vi "Write Read Visa Port Waitfor.vi"(6 "Wait for timeout (secs)":dbl=10.0, 7 "Wait for in RX":string, 8 "error in (no error)":errorcluster, 9 "Wait for read Msecs":dbl=500.0, 10 "write buffer":string, 11 "VISA Refnum in":refnum<visa-resource-name>) -> (0 "error out":errorcluster, 1 "Elapsed Time":string, 2 "read buffer":string, 3 "VISA resource name out":refnum<visa-resource-name>)   [LabVIEW 2013]
panel:
  in  "stop":bool
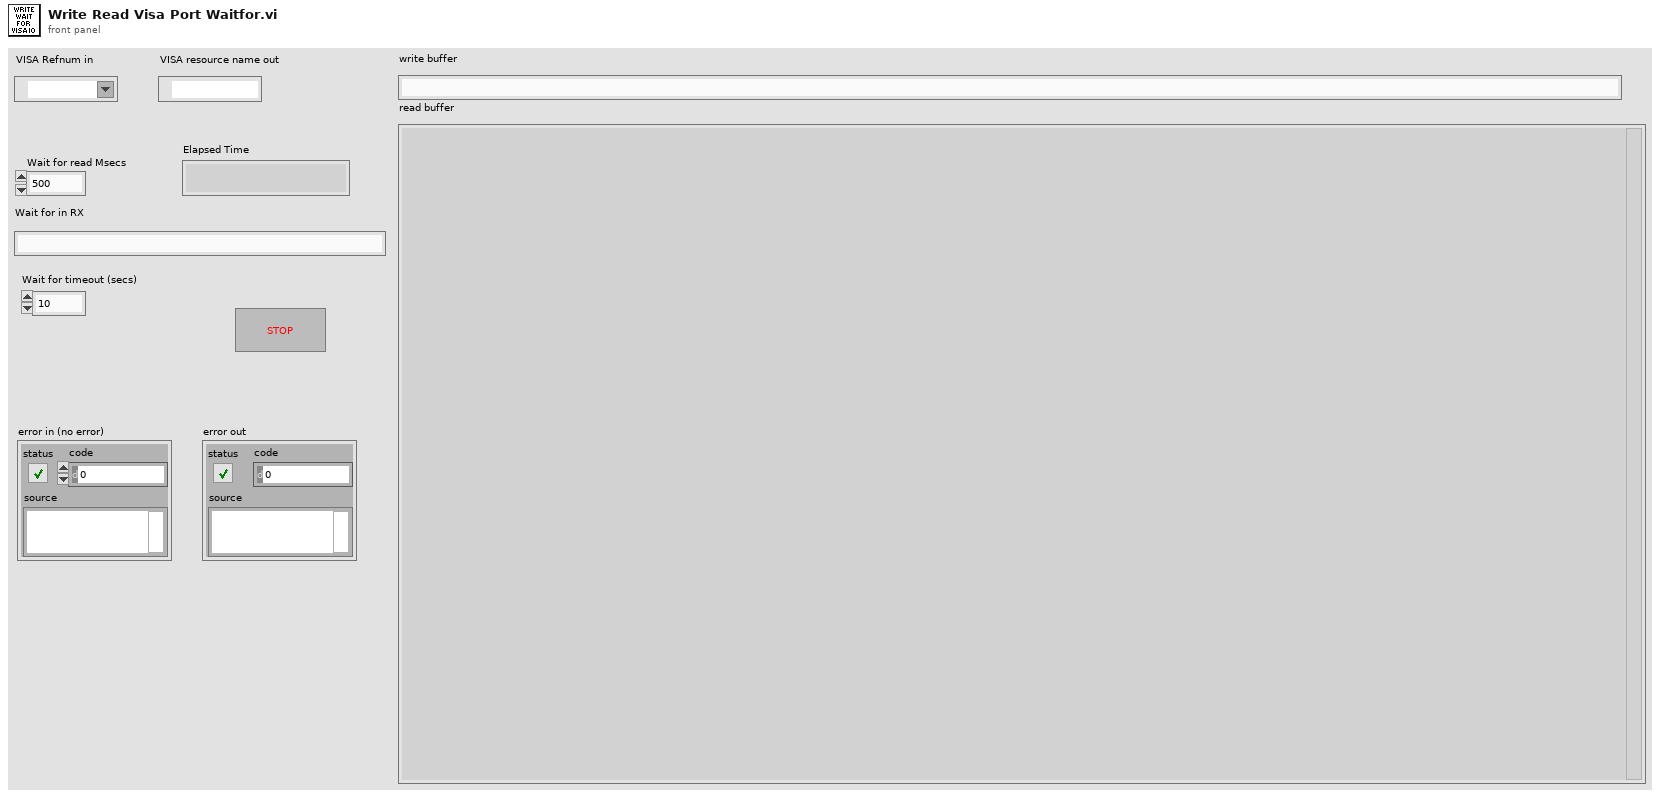
[diagram p1: front panel]
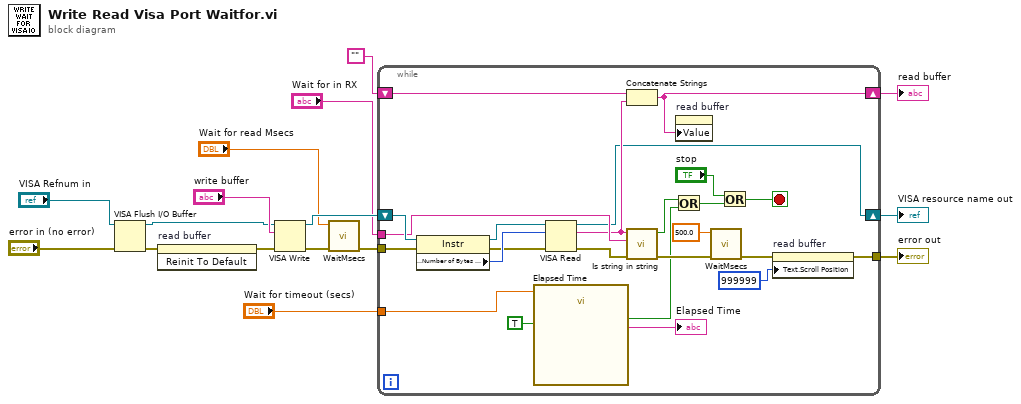
[diagram p0: block diagram]
diagram:
  n1 = VISA Flush I/O Buffer(VISA resource name="VISA Refnum in", error in (no error)="error in (no error)") -> (VISA resource name out=w3:refnum<visa-resource-name>, error out=w1:errorcluster)  [unwired: 1 in]
  n2 = invoke on="read buffer" class="Str" method="Reinit To Default"(error in=w1) -> (error out=w5:errorcluster)  [unwired: 2 in, 2 out]
  n3 = VISA Write(VISA resource name=w3, write buffer="write buffer", error in (no error)=w5) -> (VISA resource name out=w16:refnum<visa-resource-name>, error out=w15:errorcluster)  [unwired: 1 out]
  n4 = call "WaitMsecs.vi"("error in (no error)"=w15, "Wait Msecs"="Wait for read Msecs") -> ("error out"=w6:errorcluster)  [unwired: 9 in]
  n5 = while {
    tunnel: "Wait for in RX" -> [w35]
    tunnel: [w18] -> w11
    shift-right: [w25] -> w7
    shift-left: "" -> [w34]
    tunnel: "Wait for timeout (secs)" -> [w28]
    shift-right: [w26] -> w8
    shift-left: w16 -> [w37]
    tunnel: w6 -> [w24]
    stop <- w21 stop-if-true
    n6 = property class="Instr"(reference=w37, error in=w24) -> (reference out=w38:refnum<visa-resource-name>, error out=w39:errorcluster, "Serial Settings:Number of Bytes at Serial Port"=w40:u32)
    n7 = call "Elapsed Time"("Time Target (s)"=w28, "Auto Reset"=TRUE) -> ("Time has Elapsed"=w29:bool, "Elapsed Time Text"=→"Elapsed Time":string)  [unwired: 10 in, 6 out]
    n8 = VISA Read(VISA resource name=w38, byte count=w40, error in (no error)=w39) -> (VISA resource name out=w26:refnum<visa-resource-name>, read buffer=w27:string, error out=w36:errorcluster)  [unwired: 1 out]
    n9 = Concatenate Strings(w34, w27) -> (w25:string)
    n10 = call "Is string in string.vi"("error in (no error)"=w36, "Search for string"=w35, "String buffer"=w27) -> ("error out"=w33:errorcluster, "In string?"=w30:bool)  [unwired: 7 in]
    n11 = Or(x=w30, y=w29) -> (x .or. y?=w22:bool)
    n12 = property on="read buffer" class="Str"("Value"=w25) -> ()  [unwired: 2 in, 2 out]
    n13 = call "WaitMsecs.vi"("error in (no error)"=w33, "Wait Msecs"=500.0) -> ("error out"=w19:errorcluster)  [unwired: 9 in]
    n14 = Or(x="stop", y=w22) -> (x .or. y?=w21:bool)
    n15 = property on="read buffer" class="Str"(error in=w19, "Text.Scroll Position"=u32 999999) -> (error out=w18:errorcluster)  [unwired: 1 in, 1 out]
  }
  "error out" <- w11
  "VISA resource name out" <- w8
  "read buffer" <- w7
